vi "Handle Command.vi"(8 "error in":errorcluster, 10 "CMD in":refnum<class "Update Filter State CMD.lvclass">, 11 "Object In":refnum<class>) -> (0 "error out":errorcluster, 1 "Command Successful?":bool, 2 "CMD out":refnum<class "Update Filter State CMD.lvclass">, 3 "Object Out":refnum<class>)   [LabVIEW 2014, in "ePAS Library.lvlib" / "Update Filter State CMD.lvclass"]
doc: "This VI will contain the code used to actually execute the request. If the request is successful, this will be indicated by the boolean output <b>Command Successful?</b>. The boolean output can then be used by the <b>Command Reply</b> which sends a reply if the reply queue is valid."
uses:
  Update Filter State CMD.lvclass
  reusable/PAS/Main/PAS.lvclass
  reusable/PAS/Data/Main/PAS Data.lvclass
  reusable/Instrument/Instrument.lvclass/Instrument.ctl
  Update Filter State CMD.lvclass/Update Filter State CMD.ctl
  reusable/Instrument/Read Data.vi
  reusable/Instrument/Read Log Session.vi
  reusable/Instrument/Write Data.vi
  reusable/PAS/Data/Main/Write filter.vi
  reusable/Data/Data.lvclass
  <userlib>/_Session Fwk/Session - Root.lvclass
  reusable/Session APIs/Session Log/System Log.lvclass
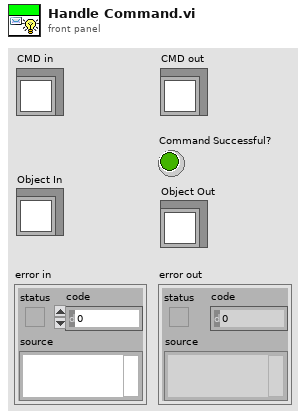
[diagram p1: front panel]
types:
  T1 = typedef "Session - Root.lvclass/Session Handle.ctl" = refnum<data-value>
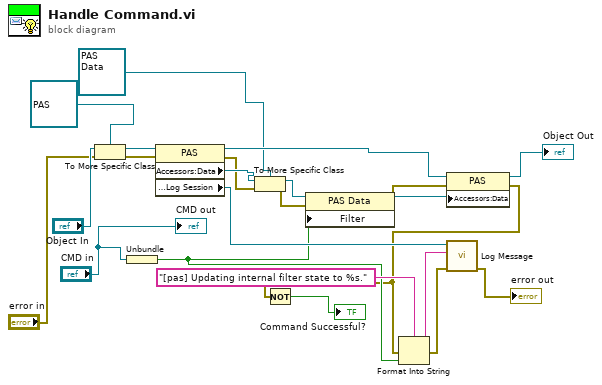
[diagram p0: block diagram]
diagram:
  n1 = To More Specific Class(target class=refnum<class "PAS.lvclass"> refnum ("PAS Library.lvlib:PAS"), reference="Object In", error in="error in") -> (specific class reference=w22:refnum<class "PAS.lvclass">, error out=w16:errorcluster)
  n2 = Unbundle("CMD in") -> (w8:bool)
  n3 = property class="PAS"(reference=w22, error in=w16) -> (reference out=w7:refnum<class "PAS.lvclass">, error out=w17:errorcluster, "Accessors:Data"=w21:refnum<class "Data.lvclass">, "Accessors:Log Session"=w14:T1)
  n4 = To More Specific Class(target class=refnum<class "PAS Data.lvclass"> refnum ("PAS Library.lvlib:PAS Data"), reference=w21, error in=w17) -> (specific class reference=w20:refnum<class "PAS Data.lvclass">, error out=w18:errorcluster)
  n5 = property class="PAS Data"(reference=w20, error in=w18, "Filter"=w8) -> (reference out=w5:refnum<class "PAS Data.lvclass">, error out=w4:errorcluster)
  n6 = property class="PAS"(reference=w7, error in=w4, "Accessors:Data"=w5) -> (reference out=→"Object Out":refnum<class "PAS.lvclass">, error out=w3:errorcluster)
  n7 = Not(x=w3) -> (.not. x?=→"Command Successful?":bool)
  n8 = Format Into String(format string="[pas] Updating internal filter state to %s.", error in=w3, w8) -> (resulting string=w11:string, error out=w12:errorcluster)  [unwired: 1 in]
  n9 = call "Log Message.vi"("error in"=w12, "MSG In"=w11, "session in"=w14) -> ("error out"=→"error out":errorcluster)  [unwired: 7 in, 1 out]
  "CMD out" <- "CMD in"
